vi "Balls.vi"() -> ()   [LabVIEW 2018]
panel:
  in  "Stop (F)":bool
  out "Image Out":T1(plugin-control)
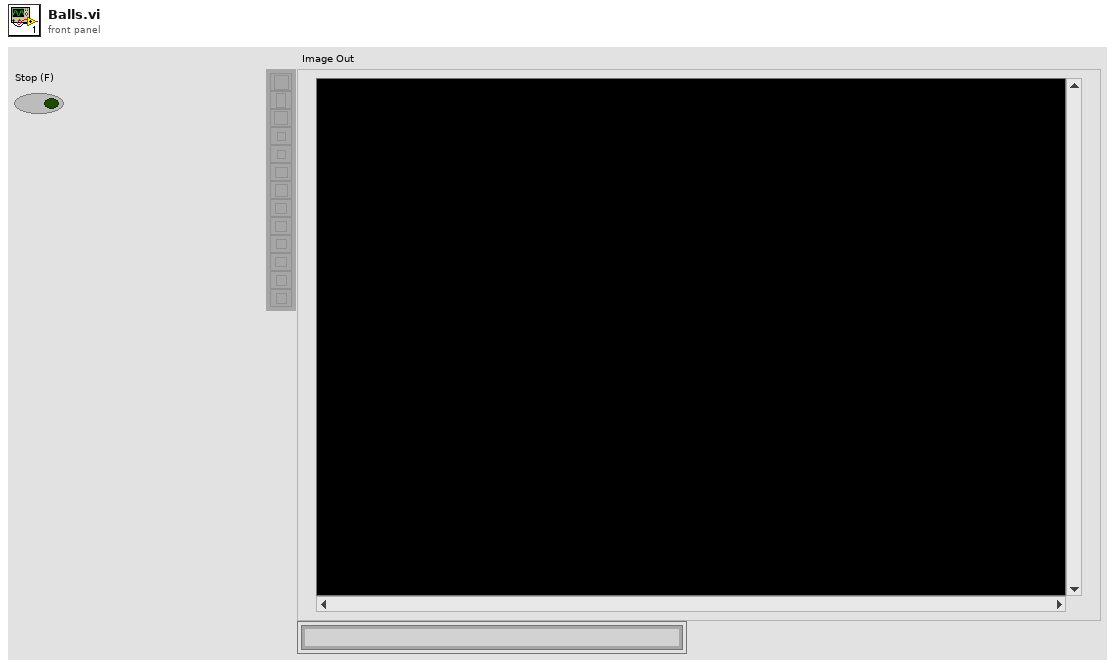
[diagram p1: front panel]
types:
  T1 = typedef "IMAQ Image.ctl" = refnum<image>
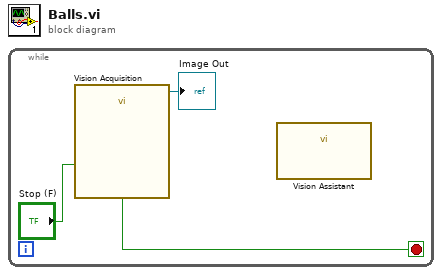
[diagram p0: block diagram]
diagram:
  n1 = while {
    stop <- w1 stop-if-true
    n2 = call "Vision Acquisition"("Stop (F)"="Stop (F)") -> ("Image Out"=→"Image Out":T1, "Stopped"=w1:bool)  [unwired: 24 in, 1 out]
    n3 = call "Vision Assistant"() -> ()  [unwired: 12 in]
  }
